vi "Catch Nested Value Update.vi"(8 "error in (no error)":errorcluster, 10 "Nested Value Update Msg":refnum<class "Nested Value Update Msg.lvclass">, 11 "Popup ViewManager ViewModel In":refnum<class "Popup ViewManager ViewModel.lvclass">) -> (0 "error out":errorcluster, 3 "Popup ViewManager ViewModel Out":refnum<class "Popup ViewManager ViewModel.lvclass">)   [LabVIEW 2017, in "Popup ViewManager ViewModel.lvclass"]
doc: "<License>\nCopyright © 2017 Composed Systems, LLC | All rights reserved\nwww.composed.io\n\nAuthor: Ethan Stern <ethan.stern@composed.io>\n\nThis software is provided \"AS IS\" WITHOUT WARRANTIES, either express or implied, AND IS FOR EDUCATIONAL PURPOSES ONLY.\n</License>"
uses:
  <vilib>/gpm_packages/@cs/popup-viewmanager/Example/ViewModel/Popup ViewManager ViewModel.lvclass
  C:/Program Files/National Instruments/LabVIEW 2017/vi.lib/gpm_packages/@cs/mva-viewable/Source/IViewModel/IViewModel/IViewModel.lvclass
  <vilib>/gpm_packages/@cs/mva-viewable/Source/IViewable/IViewable Messages/Catch Nested Value Change Msg/Nested Value Update Msg.lvclass
  <vilib>/gpm_packages/@cs/mva-viewable/Source/IViewable/IViewable Messages/Catch Nested Value Change Msg/Nested Value Update Msg.lvclass/Nested Value Update Msg.ctl
  <vilib>/gpm_packages/@cs/mva-core/Source/IObserver/IObserver/IObserver.lvclass/IObserver.ctl
  <vilib>/gpm_packages/@cs/mva-viewable/Source/IViewModel/IViewModel/IViewModel.lvclass/IViewModel.ctl
  <vilib>/gpm_packages/@cs/mva-core/Source/IMediator/PublishRequest/PublishRequest.lvclass/PublishRequest.ctl
  <vilib>/gpm_packages/@cs/mva-core/Source/IMediator/IMediator Messages/Publish Msg/Publish Msg.lvclass/Publish Msg.ctl
  <vilib>/gpm_packages/@cs/actor-framework-messages/Source/RoundTripMessage/RoundTripMessage.lvclass/RoundTripMessage.ctl
  <vilib>/ActorFramework/Message Enqueuer/Message Enqueuer.lvclass/Message Enqueuer.ctl
  <vilib>/gpm_packages/@cs/mva-core/Source/IMediator/IMediator Messages/Publish Msg/Send Pre-Addressed Publish.vi
  <vilib>/gpm_packages/@cs/mva-core/Source/IObserver/IObserver/Read Unique ID.vi
  <vilib>/gpm_packages/@cs/mva-core/Source/IMediator/PublishRequest/Pack Publish Request.vi
  <vilib>/gpm_packages/@cs/actor-framework-messages/Source/RoundTripMessage/Return Round-Trip Message.vi
  <vilib>/ActorFramework/Message Enqueuer/Enqueue.vi
  <vilib>/gpm_packages/@cs/mva-viewable/Source/IViewModel/IViewModel/IViewModel.lvclass
  C:/Program Files/National Instruments/LabVIEW 2017/vi.lib/gpm_packages/@cs/mva-core/Source/IObserver/IObserver/IObserver.lvclass
  <vilib>/gpm_packages/@cs/mva-core/Source/IMediator/IMediator Messages/Publish Msg/Publish Msg.lvclass
  C:/Program Files/National Instruments/LabVIEW 2017/vi.lib/gpm_packages/@cs/actor-framework-messages/Source/RoundTripMessage/RoundTripMessage.lvclass
  <vilib>/gpm_packages/@cs/actor-framework-messages/Source/RoundTripMessage/RoundTripMessage.lvclass
  C:/Program Files/National Instruments/LabVIEW 2017/vi.lib/ActorFramework/Message/Message.lvclass
  <vilib>/Utility/error.llb/Error Cluster From Error Code.vi
  <vilib>/ActorFramework/Message Priority Queue/Priority Enqueue.vi
  <vilib>/gpm_packages/@cs/mva-core/Source/IMediator/PublishRequest/PublishRequest.lvclass
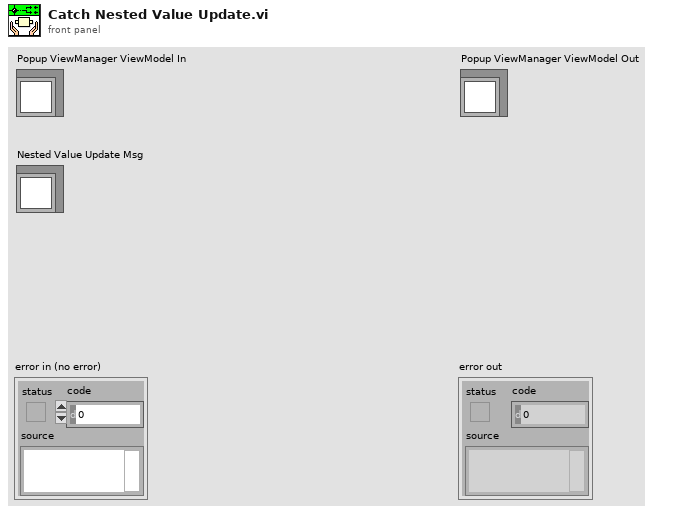
[diagram p1: front panel]
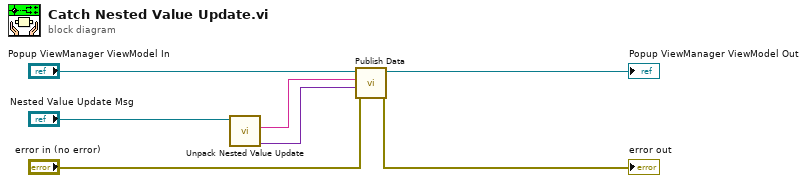
[diagram p0: block diagram]
diagram:
  n1 = call <vilib>:"Unpack Nested Value Update.vi"("Nested Value Update Msg"="Nested Value Update Msg") -> ("Value"=w1:variant, "Datum Name"=w2:string)  [unwired: 8 in, 1 out]
  n2 = call <vilib>:"Publish Data.vi"("error in (no error)"="error in (no error)", "Data to Publish"=w1, "Datum Name"=w2, "IViewModel In"="Popup ViewManager ViewModel In") -> ("error out"=→"error out":errorcluster, "IViewModel Out"=→"Popup ViewManager ViewModel Out":refnum<class "Popup ViewManager ViewModel.lvclass">)  [unwired: 6 in]
